vi "Prema Get Volts.vi"(8 "error in":errorcluster, 11 "VISA resource name":refnum<visa-resource-name>) -> (0 "error out":errorcluster, 1 "data string out":string, 2 "value":dbl, 3 "VISA resource name out":refnum<visa-resource-name>)   [LabVIEW 2021]
uses:
  GPIB/VISA  Send Receive.vi
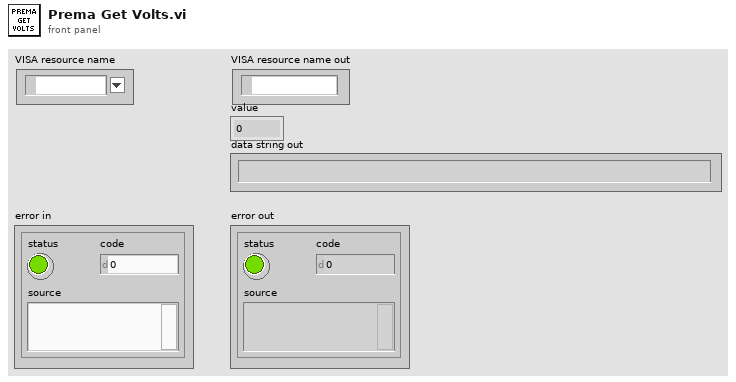
[diagram p1: front panel]
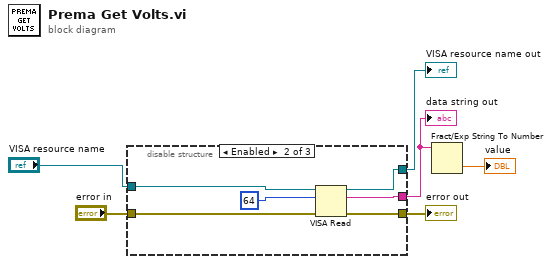
[diagram p0: block diagram]
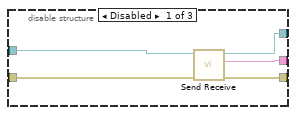
[diagram p2: hidden frame]
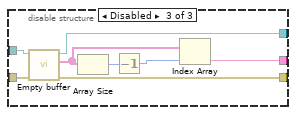
[diagram p3: hidden frame]
diagram:
  n1 = disable-structure shown="Enabled" {
    disable-tunnel: "VISA resource name" -> [w11 w13 w25]
    disable-tunnel: "error in" -> [w10 w17 w24]
    disable-tunnel: [w9 w16 w23] -> w4
    disable-tunnel: [w8 w14 w22] -> w3
    disable-tunnel: [w7 w15 w18] -> w2
    frame Disabled {
      n2 = call-poly "Send Receive.vi"("error in (no error)"=w10, "VISA Resource Name"=w11) -> ("error out"=w9:errorcluster, "data string out"=w7:string, "VISA Resource Name Out"=w8:refnum<visa-resource-name>)  [unwired: 7 in]
    }
    frame Enabled {
      n3 = VISA Read(VISA resource name=w13, byte count=u32 64, error in (no error)=w17) -> (VISA resource name out=w14:refnum<visa-resource-name>, read buffer=w15:string, error out=w16:errorcluster)  [unwired: 1 out]
    }
    frame Disabled {
      n4 = call "Empty buffer.vi"("Error In"=w24, "VISA resource name"=w25) -> ("Error Out"=w23:errorcluster, "Buffer content"=w19:string[], "VISA resource name out"=w22:refnum<visa-resource-name>)  [unwired: 7 in]
      n5 = Array Size(array=w19) -> (size(s)=w21:i32)
      n6 = Decrement(x=w21) -> (x-1=w20:i32)
      n7 = Index Array(array=w19, index=w20) -> (element=w18:string)
    }
  }
  "error out" <- w4
  "VISA resource name out" <- w3
  "data string out" <- w2
  n8 = Fract/Exp String To Number(string=w2) -> (number=→"value":dbl)  [unwired: 3 in, 1 out]
